vi "GUI_CapSpec.vi"() -> ()   [LabVIEW 2011]
uses:
  GUI_Template/GUI_master/tcp_new_data_event.ctl
  GUI_Template/GUI_master/tcp new data cluster.ctl
panel:
  out "Waveform Graph":dbl[](graph)
  out "Numeric":i32
  out "image::1":T1(plugin-control) caption="StagingCapSpec"
  in  "stop":bool
  in  "GUIdevice 1":string="StagingCapSpec"
  out "tcp data event":T2
  out "error IO 2":errorcluster
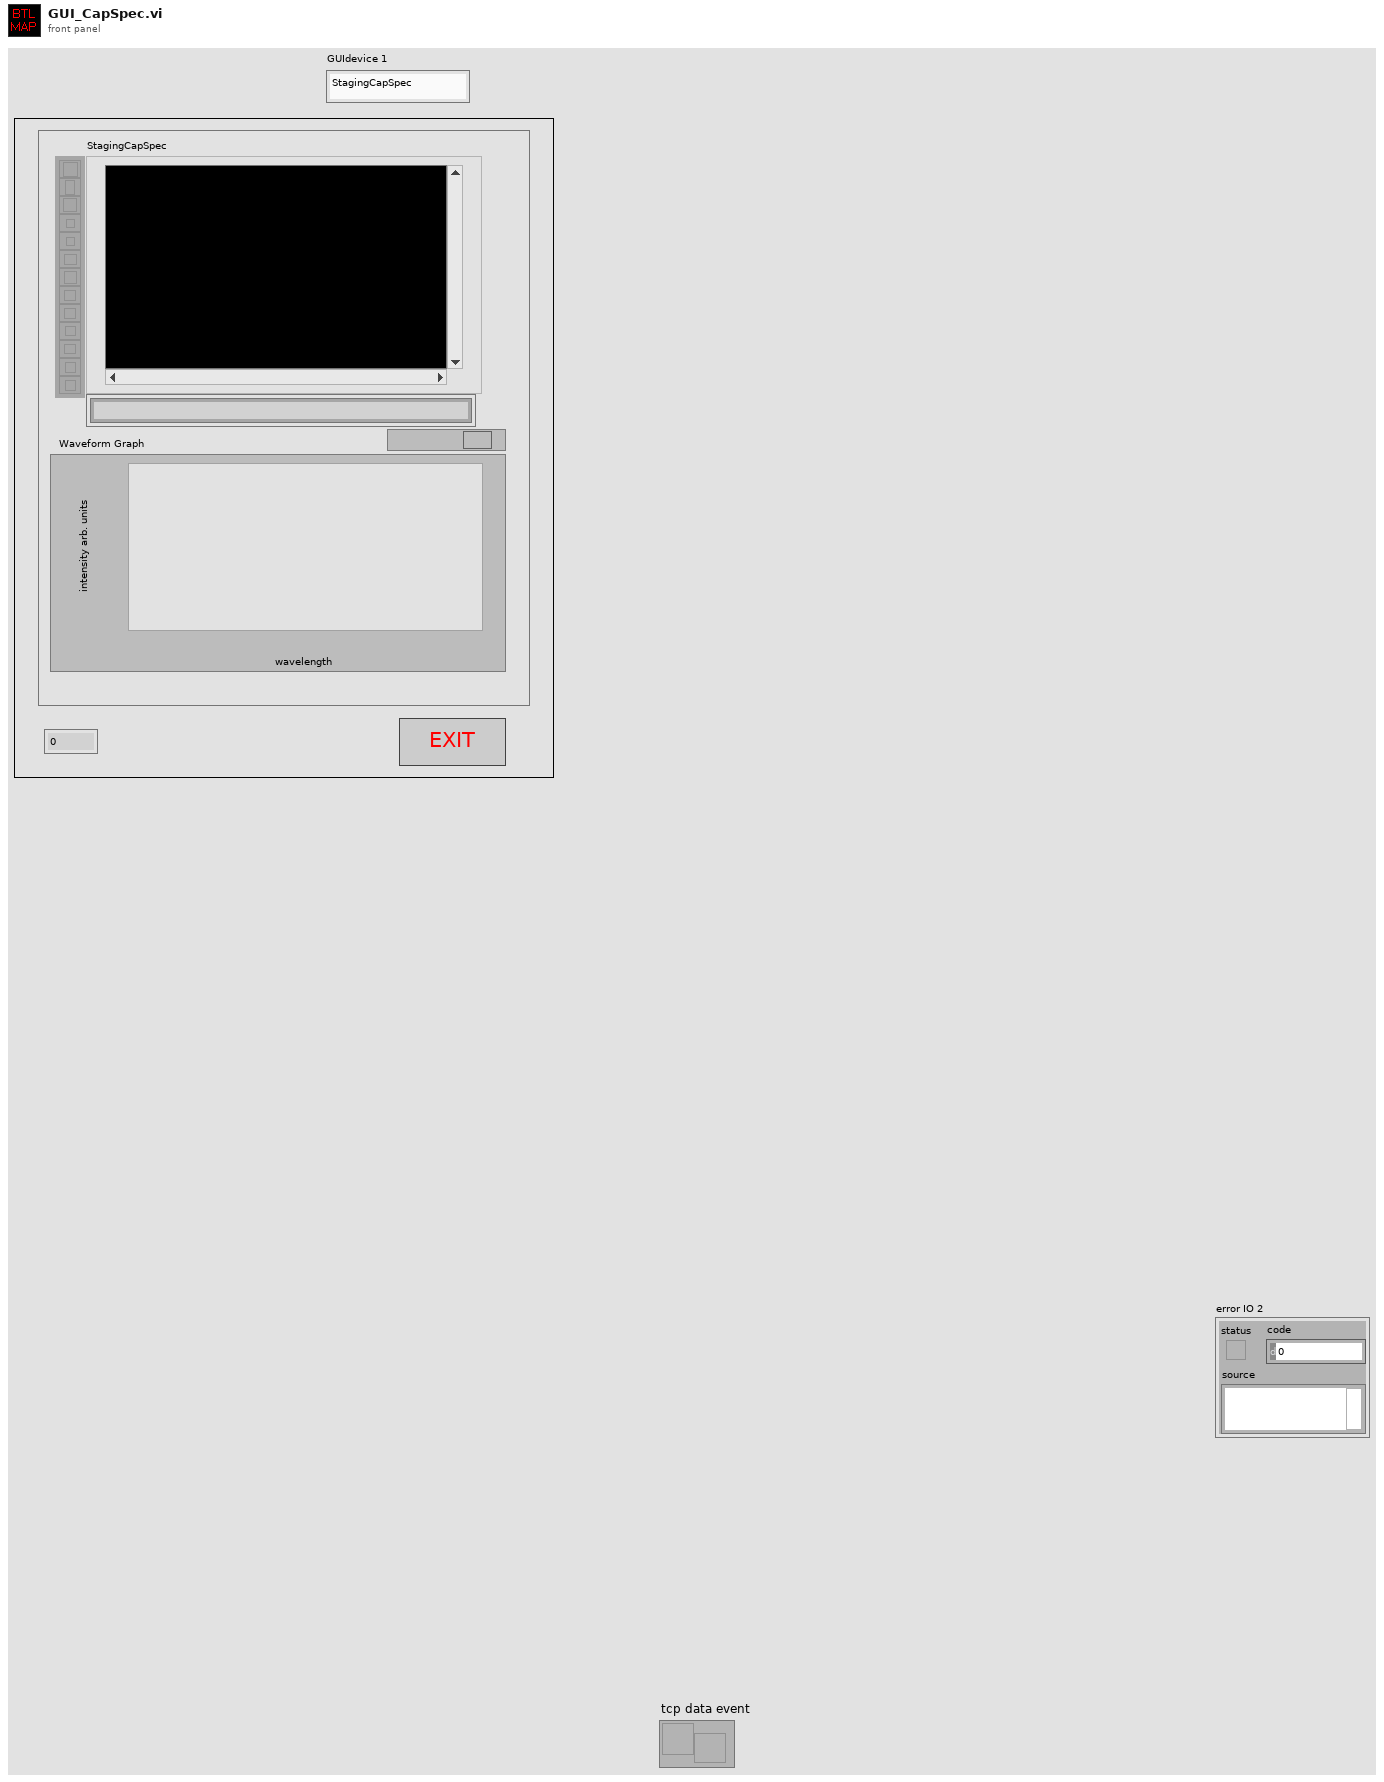
[diagram p1: front panel]
types:
  T1 = typedef "IMAQ Image.ctl" = refnum<image>
  T2 = typedef "tcp_new_data_event.ctl" = refnum<user-event>
  T3 = typedef "tcp new data cluster.ctl" = cluster{"EventEnum":enum16{"new data", "connection status update"}, "Device name":string}
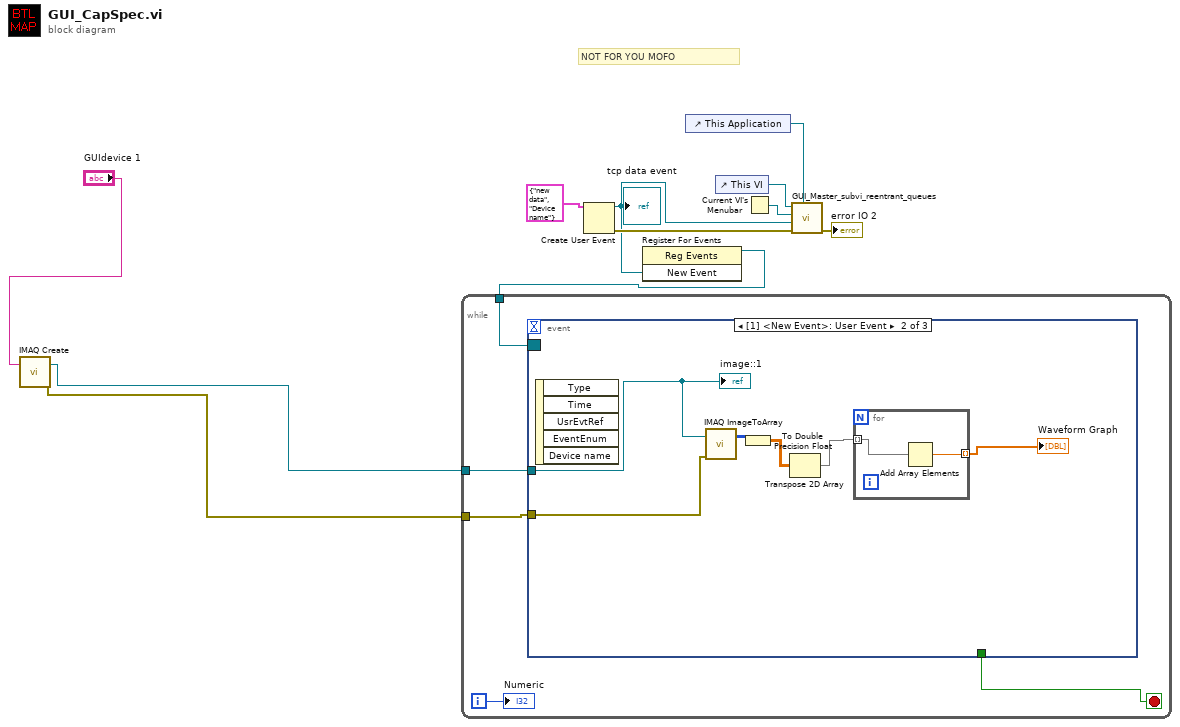
[diagram p0: block diagram]
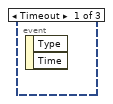
[diagram p2: hidden frame]
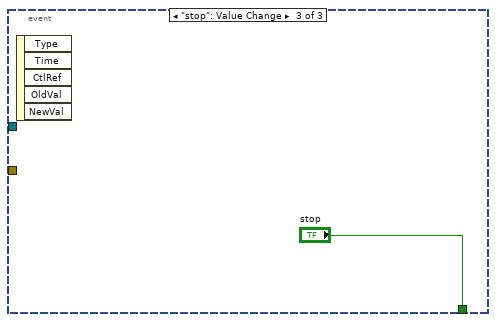
[diagram p3: hidden frame]
diagram:
  # "NOT FOR YOU MOFO"
  n1 = call "IMAQ Create"("Image Name"="GUIdevice 1") -> ("New Image"=w2:T1, "error out"=w1:errorcluster)  [unwired: 4 in]
  n2 = Create User Event(user event datatype=T3 {"EventEnum"=enum."new data", "Device name"="Device name"} ("New Event")) -> (user event=w6:refnum<user-event>, error out=w7:errorcluster)  [unwired: 1 in]
  "tcp data event" <- w6
  n3 = register-events(w6) -> (reference out=w4:refnum<event-registration>)  [unwired: 2 in, 1 out]
  n4 = while {
    tunnel: w4 -> [w16]
    tunnel: w2 -> [w14]
    tunnel: w1 -> [w12]
    i -> [w13]
    stop <- w15 stop-if-true
    n5 = event shown="[1] <New Event>: User Event" {
      selector: w16 -> [_ _ _]
      dyn-events: _ -> [_ _ _]
      timeout: _ -> [_ _ _]
      tunnel: [_ _ "stop"] -> w15
      tunnel: w14 -> [_ w17 _]
      tunnel: w12 -> [_ w22 _]
      event Timeout {
        n6 = event-data() -> ()  [unwired: 1 in, 2 out]
      }
      event User Event {
        n7 = event-data() -> ()  [unwired: 1 in, 5 out]
        n8 = call "IMAQ ImageToArray"("error in (no error)"=w22, "Image"=w17) -> ("Image Pixels (I16)"=w21:i16[][])  [unwired: 2 in, 4 out]
        n9 = To Double Precision Float(number=w21) -> (double precision float=w19:dbl[][])
        n10 = Transpose 2D Array(2D array=w19) -> (transposed array=w18:dbl[][])
        n11 = for {
          tunnel: w18 -> [w24] mode=indexing
          tunnel: [w23] -> w20 mode=indexing
          n12 = Add Array Elements(numeric array=w24) -> (sum=w23:dbl)
        }
        "Waveform Graph" <- w20
        "image::1" <- w17
      }
      event "stop": Value Change {
        n13 = event-data() -> ()  [unwired: 1 in, 5 out]
      }
    }
    "Numeric" <- w13
  }
  n14 = control-ref of="This Application"() -> (w5:refnum<vi>)
  n15 = control-ref of="This VI"() -> (w10:refnum<vi>)
  n16 = Current VI's Menubar() -> (w9:refnum<k9>)
  n17 = call "GUI_Master_subvi_reentrant_queues.vi"("This Application"=w5, "error in (no error)"=w7, "tcp data event"=w6, "Caller menu reference"=w9, "Caller VI ref"=w10) -> ("error out"=→"error IO 2":errorcluster)  [unwired: 6 in]
